vi "Statistical Analysis.vi"(8 "error in (no error)":cluster{"状态":bool, "代码":i32, "源":string} caption="错误输入（无错误）", 11 "图形数据输入":T1) -> (0 "error out":cluster{"状态":bool, "代码":i32, "源":string} caption="错误输出", 3 "图形数据输出":T1)   [LabVIEW 2013]
doc: "计算输入数据中每个波形的一些基本统计量（均值、RMS、最小值、最大值、峰峰值，以及频率），并输出注释。"
uses:
  controls/Graph Data.ctl
  <vilib>/Utility/miscctls.llb/LVAnnotationListTypeDef.ctl
  <vilib>/Utility/miscctls.llb/LVCursorListTypeDef.ctl
panel:
  # "（向上滚动可查看大型数据输入/输出簇）"
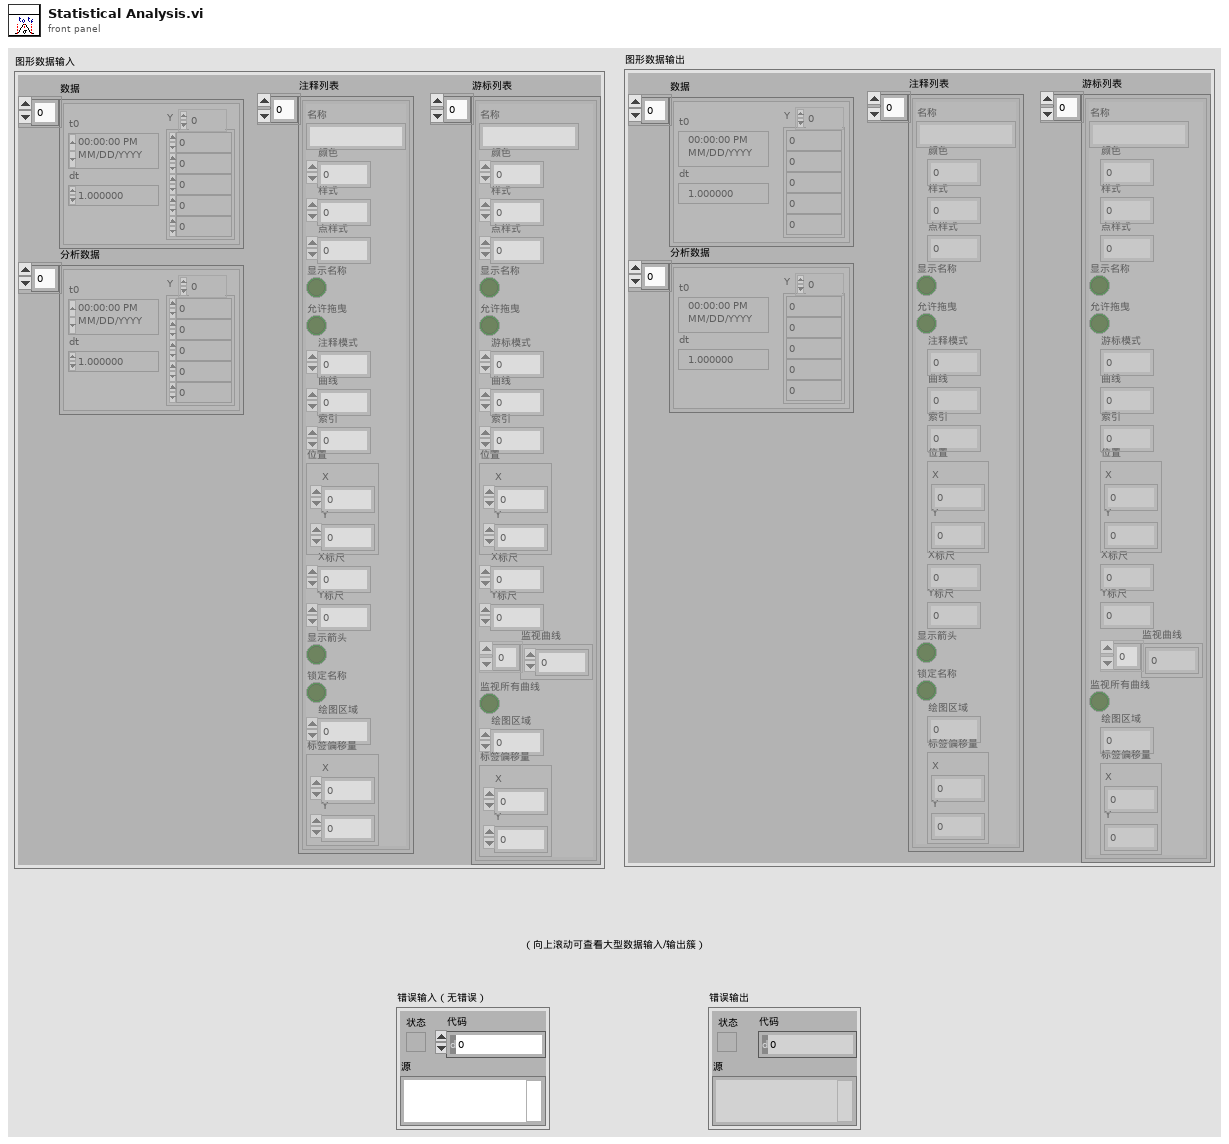
[diagram p1: front panel]
types:
  T1 = typedef "Graph Data.ctl" = cluster{"数据":waveform(dbl)[], "注释列表":T2, "游标列表":T3, "分析数据":waveform(dbl)[]}
  T2 = typedef "LVAnnotationListTypeDef.ctl" = cluster{"Name":string, "Color":u32, "Style":u8, "Point Style":u8, "Name Visible":bool, "Allow Drag":bool, "Annotation Mode":u32, "Plot":i32, "Index":i32, "Position":cluster{"X":dbl, "Y":dbl}, "X Scale":u32, "Y Scale":u32, "Show Arrow":bool, "Lock Name":bool, "Plot Area":i32, "Label Offset":cluster{"X":dbl, "Y":dbl}}[]
  T3 = typedef "LVCursorListTypeDef.ctl" = cluster{"Name":string, "Color":u32, "Style":u8, "Point Style":u8, "Name Visible":bool, "Allow Drag":bool, "Cursor Mode":u32, "Plot":i32, "Index":i32, "Position":cluster{"X":dbl, "Y":dbl}, "X Scale":u32, "Y Scale":u32, "Watch Plots":i32[], "Watch All Plots":bool, "Plot Area":i32, "Label Offset":cluster{"X":dbl, "Y":dbl}}[]
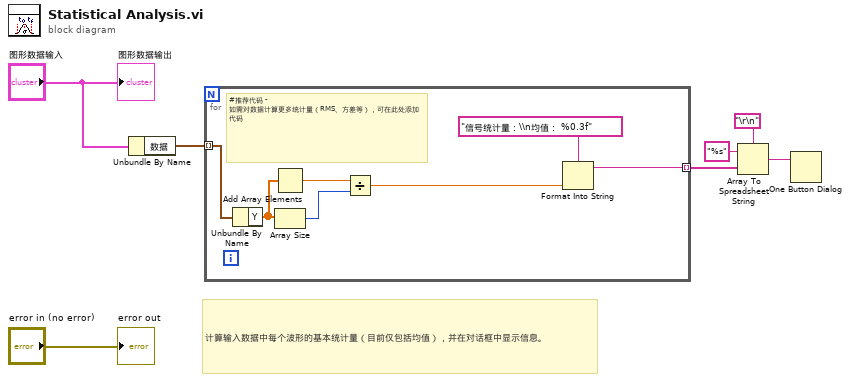
[diagram p0: block diagram]
diagram:
  # "计算输入数据中每个波形的基本统计量（目前仅包括均值），并在对话框中显示信息。"
  n1 = Unbundle By Name("图形数据输入") -> ("数据"=w7:waveform(dbl)[])
  n2 = for {
    tunnel: w7 -> [w14] mode=indexing
    tunnel: [w9] -> w4 mode=indexing
    # "#推荐代码 - 如需对数据计算更多统计量（RMS、方差等），可在此处添加代码"
    n3 = Unbundle By Name(w14) -> ("Y"=w10:dbl[])
    n4 = Add Array Elements(numeric array=w10) -> (sum=w13:dbl)
    n5 = Array Size(array=w10) -> (size(s)=w11:i32)
    n6 = Divide(x=w13, y=w11) -> (x/y=w12:dbl)
    n7 = Format Into String(format string="信号统计量：\\n均值： %0.3f" ("Signal Statistics"), w12) -> (resulting string=w9:string)  [unwired: 2 in, 1 out]
  }
  n8 = Array To Spreadsheet String(delimiter (Tab)="\r\n", array=w4, 3:"%s" ("format string")) -> (spreadsheet string=w1:string)
  n9 = One Button Dialog(message=w1) -> ()  [unwired: 1 in, 1 out]
  "error out" <- "error in (no error)"
  "图形数据输出" <- "图形数据输入"
